vi "MoveWindow.vi"() -> ()   [LabVIEW 2020]
uses:
  C:/Users/dzoni/Documents/NJ/Playground/LV/WinAPI/DLL/WinAPI.dll
  DLL/WinAPI.dll
  System.Windows.Forms
  System.Drawing
panel:
  out "Width":i32
  out "Height":i32
  out "Bottom":i32[](array[numeric])
  out "Height":i32[](array[numeric])
  out "Y":i32[](array[numeric])
  out "X":i32[](array[numeric])
  out "DevIDs":string[](array[string])
  out "Primary":bool[](array[boolean])
  out "Left":i32[](array[numeric])
  out "Right":i32[](array[numeric])
  out "Width":i32[](array[numeric])
  out "Top":i32[](array[numeric])
  in  "Move":bool
  out "MoveWindowByName":bool
  in  "Y":i32
  in  "X":i32
  in  "EXE (T) or VI (F)":bool
  in  "EXE name":string
  out "error out":errorcluster
  out "VI Name":string
  out "NumOfMon":i32
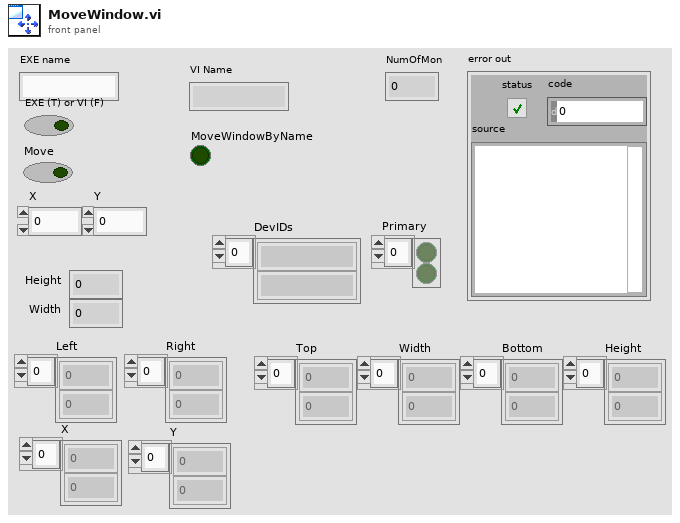
[diagram p1: front panel]
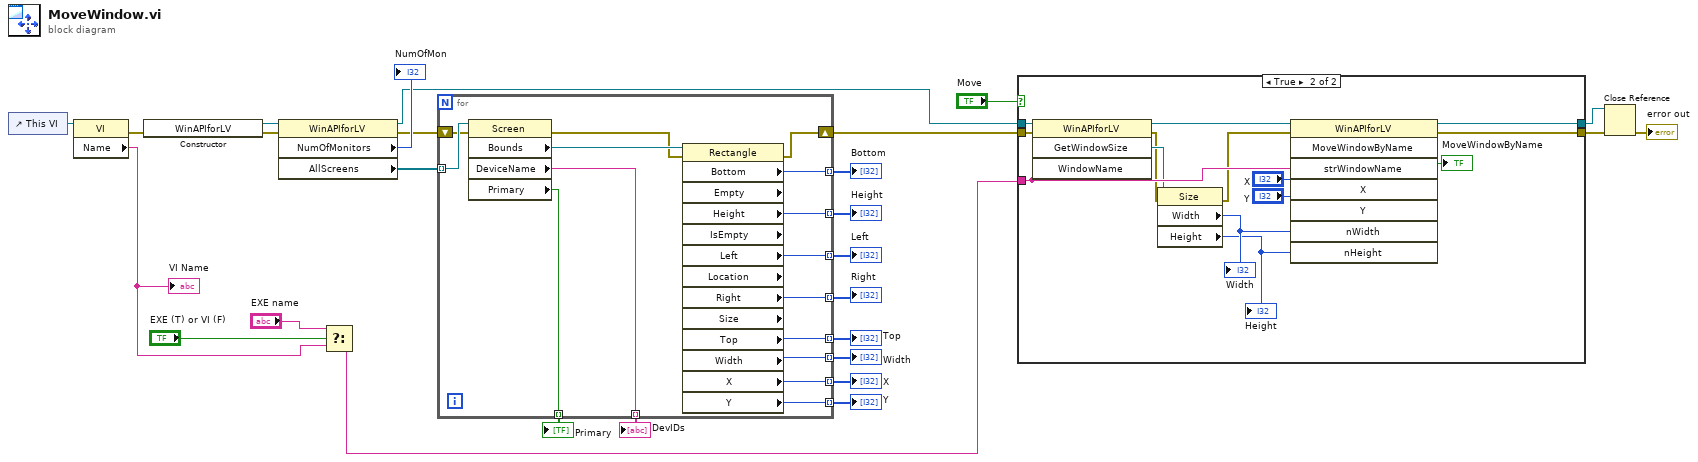
[diagram p0: block diagram]
diagram:
  n1 = control-ref of="This VI"() -> (w26:refnum<vi>)
  n2 = property class="VI"(reference=w26) -> (error out=w17:errorcluster, "Name"=w22:string)  [unwired: 1 in, 1 out]
  "VI Name" <- w22
  n3 = constructor class="WinAPIforLV"(error in=w17) -> (reference out=w21:refnum<k24>, error out=w19:errorcluster)  [unwired: 2 in, 1 out]
  n4 = property class="WinAPIforLV"(reference=w21, error in=w19) -> (reference out=w12:refnum<k24>, error out=w14:errorcluster, "NumOfMonitors"=→"NumOfMon":i32, "AllScreens"=w11:refnum<k24>[])
  n5 = Select(t="EXE name", s="EXE (T) or VI (F)", f=w22) -> (s? t:f=w16:string)
  n6 = for {
    tunnel: w11 -> [w38] mode=indexing
    shift-right: [w30] -> w13
    shift-left: w14 -> [w32]
    tunnel: [w42] -> w10 mode=indexing
    tunnel: [w41] -> w9 mode=indexing
    tunnel: [w40] -> w8 mode=indexing
    tunnel: [w39] -> w7 mode=indexing
    tunnel: [w29] -> w6 mode=indexing
    tunnel: [w28] -> w5 mode=indexing
    tunnel: [w36] -> w4 mode=indexing
    tunnel: [w35] -> w2 mode=indexing
    tunnel: [w34] -> w1 mode=indexing
    tunnel: [w33] -> w3 mode=indexing
    n7 = property class="Screen"(reference=w38, error in=w32) -> (error out=w31:errorcluster, "Bounds"=w37:refnum<k24>, "DeviceName"=w28:string, "Primary"=w29:bool)  [unwired: 1 out]
    n8 = property class="Rectangle" props=["Bottom", "Empty", "Height", "IsEmpty", "Left", "Location", "Right", "Size", "Top", "Width", "X", "Y"](reference=w37, error in=w31) -> (error out=w30:errorcluster, "Bottom"=w34:i32, "Height"=w35:i32, "Left"=w39:i32, "Right"=w40:i32, "Top"=w42:i32, "Width"=w41:i32, "X"=w36:i32, "Y"=w33:i32)  [unwired: 5 out]
  }
  "Top" <- w10
  "Width" <- w9
  "Right" <- w8
  "Left" <- w7
  "Primary" <- w6
  "DevIDs" <- w5
  "X" <- w4
  "Y" <- w3
  "Height" <- w2
  "Bottom" <- w1
  n9 = case shown="True" "Move" {
    tunnel: [w44 w58] -> w20
    tunnel: [w43 w57] -> w18
    tunnel: w16 -> [_ w53]
    tunnel: w13 -> [w43 w48]
    tunnel: w12 -> [w44 w49]
    frame False {
    }
    frame True {
      n10 = invoke class="WinAPIforLV" method="GetWindowSize"(reference=w49, error in=w48, "WindowName"=w53) -> (reference out=w47:refnum<k24>, error out=w46:errorcluster, "GetWindowSize"=w52:refnum<k24>)  [unwired: 1 in, 1 out]
      n11 = property class="Size"(reference=w52, error in=w46) -> (error out=w45:errorcluster, "Width"=w51:i32, "Height"=w50:i32)  [unwired: 1 out]
      "Height" <- w50
      "Width" <- w51
      n12 = invoke class="WinAPIforLV" method="MoveWindowByName"(reference=w47, error in=w45, "strWindowName"=w53, "X"="X", "Y"="Y", "nWidth"=w51, "nHeight"=w50) -> (reference out=w58:refnum<k24>, error out=w57:errorcluster, "MoveWindowByName"=→"MoveWindowByName":bool)  [unwired: 1 in, 5 out]
    }
  }
  n13 = Close Reference(reference=w20, error in (no error)=w18) -> (error out=→"error out":errorcluster)
